vi "Get Behavior Flags.vi"(8 "error in (no error)":errorcluster, 11 "Reference in":refnum<class "Reference.lvclass">) -> (0 "error out":errorcluster, 2 "Behavior":T1={"Children"=enum."None", "Editable"=TRUE, "XML uses />"=TRUE}, 3 "Reference out":refnum<class "Reference.lvclass">)   [LabVIEW 2023, in "VILab.lvlib" / "Reference.lvclass"]
uses:
  Reference.lvclass
  Data Item/Behavior Flags.ctl
  Data Item/Child Support.ctl
  Data Item.lvclass
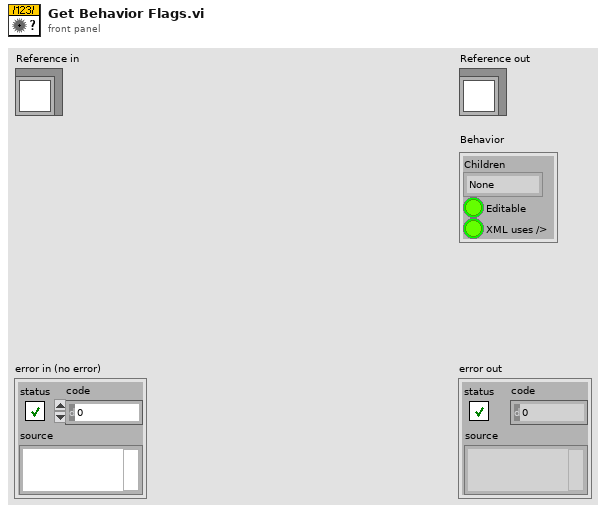
[diagram p1: front panel]
types:
  T1 = typedef "VILab.lvlib/Data Item.lvclass/Behavior Flags.ctl" = cluster{"Children":T2, "Editable":bool, "XML uses />":bool}
  T2 = typedef "VILab.lvlib/Data Item.lvclass/Child Support.ctl" = enum16{"None", "One", "At most one", "Multiple"}
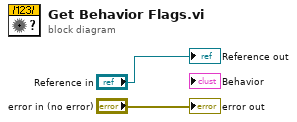
[diagram p0: block diagram]
diagram:
  "error out" <- "error in (no error)"
  "Reference out" <- "Reference in"
